vi "OE1311&OE1351_Ethernet_Query Setting.vi"(5 "Connection ID in":refnum<k5>, 7 "Timeout":u32=1000, 11 "Error in (no error)":errorcluster caption="error out（no error）") -> (1 "Input Filter":cluster{"InputCoupling":u8, "InputSource":u8} {"InputSource" items=["A", "B", "Current"]; "InputCoupling" items=["AC", "DC"]}, 2 "Sine Out":T2 {"SineOut Mode" items=["OFF", "Fixed"]}, 3 "System":T1, 6 "Connection ID out":refnum<k5>, 8 "Demodulator":T4 {"Demodulator type_7" items=["Harm", "Arb_Freq"]; "Demodulator type_6" items=["Harm", "Arb_Freq"]; "Demodulator type_5" items=["Harm", "Arb_Freq"]; "Demodulator type_4" items=["Harm", "Arb_Freq"]; "Demodulator type_3" items=["Harm", "Arb_Freq"]; "Demodulator type_2" items=["Harm", "Arb_Freq"]; "Demodulator type_1" items=["Harm", "Arb_Freq"]}, 10 "Output String":string, 12 "Reference Phase":T6 {"External Ref Trigger" items=["TTL Rising Edge", "TTL Fallling Edge", "Sine Zero Crossing"]; "Reference Source" items=["External", "Internal", "Self"]}, 13 "Sensitivity and Filter":T3={"Input Range"=2, "Time Constant(s) "=[], "Low Pass Filter Slope "=1, "Enable Sync Filter "=0} {"Enable Sync Filter" items=["OFF", "ON"]; "Low Pass Filter Slope" items=["6 dB/oct", "12 dB/oct", "18 db/oct", "24 dB/oct", "30 dB/oct", "36 dB/oct", "42 dB/oct", "48 dB/oct"]; "Input Range" items=["5 V/uA", "2 V/uA", "1 V/uA", "500 mV/nA", "200 mV/nA", "100 mV/nA", "50 mV/nA", "20 mV/nA", "10 mV/nA", "5 mV/nA", "2 mV/nA", "1 mV/nA", "500 uV/pA", "200 uV/pA", "100 uV/pA", "50 uV/pA", "20 uV/pA", "10 uV/pA", "5 uV/pA", "2 uV/pA", "1 uV/pA", "500 nV/fA", "200 nV/fA", "100 nV/fA", "50 nV/fA", "20 nV/fA", "10 nV/fA", "5 nV/fA", "2 nV/fA", "1 nV/fA"]}, 14 "Channel Out":T5={"Ch_source_1"=3, "Ch_source_2"=3, "AUX OUT1"=[], "AUX OUT2"=[], "CH1 Offset(%)"=[], "CH2 Offset(%)"=[], "CH1 Expand"=[], "CH2 Expand"=[]} {"Ch_source_2" items=["Fixed", "X", "Y", "R", "Theta", "Xh1", "Yh1", "Rh1", "Theta h1", "Xh2", "Yh2", "Rh2", "Theta h2", "Xh3", "Yh3", "Rh3", "Theta h3", "Rh4", "Xh4", "Yh4", "Theta h4", "Rh5", "Xh5", "Yh5", "Theta h5", "Rh6", "Xh6", "Yh6", "Theta h6", "Rh7", "Xh6", "Yh6", "Theta h7", "X_Noise", "Y_Noise", "Freq", "AuxIn1", "AuxIn2"]; "Ch_source_1" items=["Fixed", "X", "Y", "R", "Theta", "Xh1", "Yh1", "Rh1", "Theta h1", "Xh2", "Yh2", "Rh2", "Theta h2", "Xh3", "Yh3", "Rh3", "Theta h3", "Rh4", "Xh4", "Yh4", "Theta h4", "Rh5", "Xh5", "Yh5", "Theta h5", "Rh6", "Xh6", "Yh6", "Theta h6", "Rh7", "Xh6", "Yh6", "Theta h7", "X_Noise", "Y_Noise", "Freq", "AuxIn1", "AuxIn2"]}, 15 "Error out":errorcluster caption="error out")   [LabVIEW 2011]
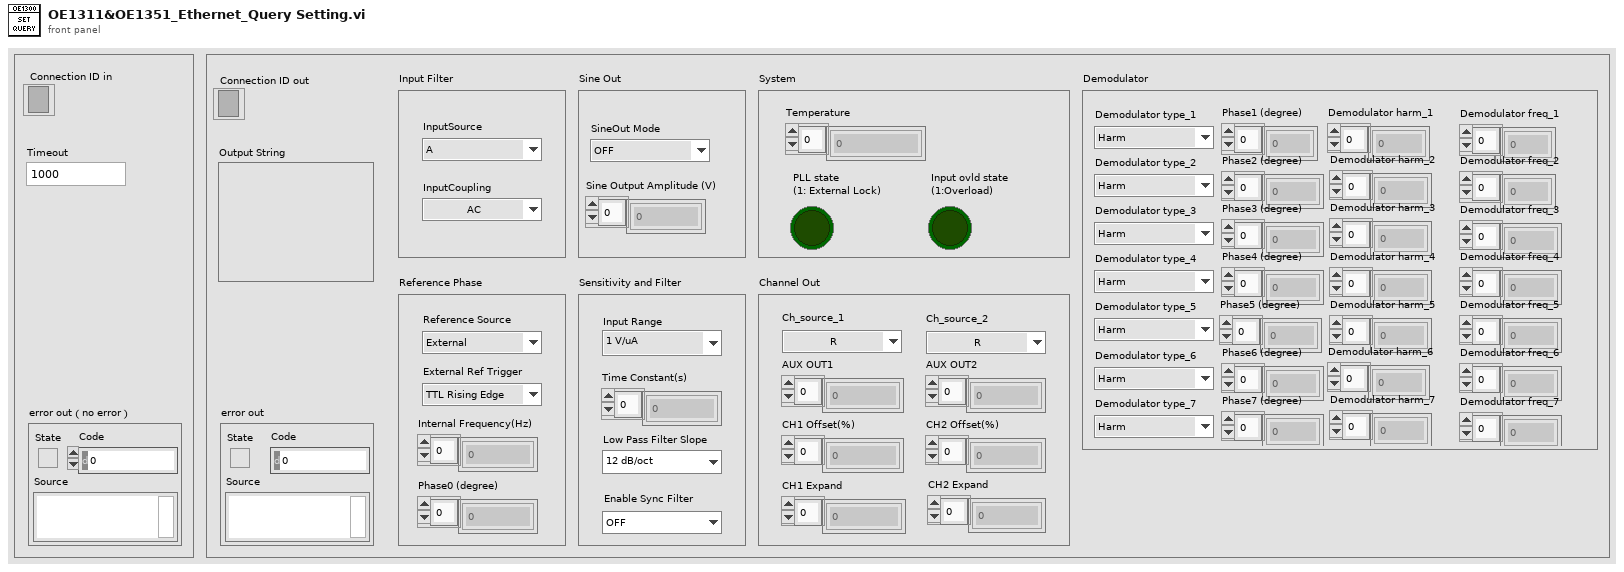
[diagram p1: front panel]
types:
  T1 = cluster{"Temperature":dbl[], "PLL state\n(1: External Lock)":bool, "Input ovld state\n(1:Overload)":bool}
  T2 = cluster{"SineOut Mode":u8, "Sine Output Amplitude (V)":dbl[]}
  T3 = cluster{"Input Range":u8, "Time Constant(s) ":dbl[], "Low Pass Filter Slope ":u8, "Enable Sync Filter ":u8}
  T4 = cluster{"Demodulator type_1":u8, "Demodulator type_2":u8, "Demodulator type_3":u8, "Demodulator type_4":u8, "Demodulator type_5":u8, "Demodulator type_6":u8, "Demodulator type_7":u8, "Phase1 (degree)":dbl[], "Phase2 (degree)":dbl[], "Phase3 (degree)":dbl[], "Phase4 (degree)":sgl[], "Phase5 (degree)":dbl[], "Phase6 (degree)":dbl[], "Phase7 (degree)":dbl[], "Demodulator harm_1":u8[], "Demodulator harm_2":u8[], "Demodulator harm_3":u8[], "Demodulator harm_4":u8[], "Demodulator harm_5":u8[], "Demodulator harm_6":u8[], "Demodulator harm_7":u8[], "Demodulator freq_1":dbl[], "Demodulator freq_2":dbl[], "Demodulator freq_3":dbl[], "Demodulator freq_4":dbl[], "Demodulator freq_5":dbl[], "Demodulator freq_6":dbl[], "Demodulator freq_7":dbl[]}
  T5 = cluster{"Ch_source_1":u8, "Ch_source_2":u8, "AUX OUT1":dbl[], "AUX OUT2":dbl[], "CH1 Offset(%)":dbl[], "CH2 Offset(%)":dbl[], "CH1 Expand":dbl[], "CH2 Expand":dbl[]}
  T6 = cluster{"Phase0 (degree)":dbl[], "Internal Frequency(Hz)":dbl[], "Reference Source":u8, "External Ref Trigger":u8}
  T7 = enum16{"ISRC", "IGND", "ICPL", "ILIN", "PHAS", "FMOD", "RSLP", "FREQ", "SWPT", "SLLM", "SULM", "SSLL", "SSLG", "STLM", "SWRM", "IRNG", "SENS", "RMOD", "OFLT", "OFSL", "SYNC", "DMOD", "HARM", "DARB", "SWVT", "SLVL", "SVLL", "SVUL", "SVSL", "SVSG", "SVTM", "SVRM", "RALL", "SNAP", "OUTP", "OAUX", "COUT", "CAUX", "COFP", "CEXP", "FPOP", "OEXP", "*IDN", "*RST", "OVLD", "INOV", "GNOV", "*PLL", "SSET", "RSET", "AGAN", "APHS", "ARSV", "ASCL", "EQCD", "EQCS", "SPED", "SRAT", "SLEN", "SSLE", "STRG", "SPRM", "STRD", "PAUS", "REST", "SPTS", "TRCA", "TEMP", "RSTU", "IHNZ", "DEQU", "SADD", "ARNG", "CSPE", "ISRCD", "IGNDD", "ICPLD", "ILIND", "PHASD", "FMODD", "RSLPD", "FREQD", "SWPTD", "SLLMD", "SULMD", "SSLLD", "SSLGD", "STLMD", "SWRMD", "SENSD", "RMODD", "OFLTD", "OFSLD", "SYNCD", "HARMD", "EQCDD", "EQCSD", "SNAPD", "OUTPD", "SWVTD", "SLVLD", "SVLLD", "SVULD", "SVSLD", "SVSGD", "SVTMD", "SVRMD", "SVDCD", "ARSVD", "AGAND", "APHSD", "ASCLD", "FPOPD", "CAUXD", "OEXPD", "SPEDD", "SRATD", "SLEND", "SSLED", "STRGD", "SPRMD", "STRDD", "PAUSD", "RESTD", "SPTSD", "TRCAD", "*IDND", "*RSTD", "INOVD", "GNOVD", "*PLLD", "SSETD", "RSETD", "RALLD"}
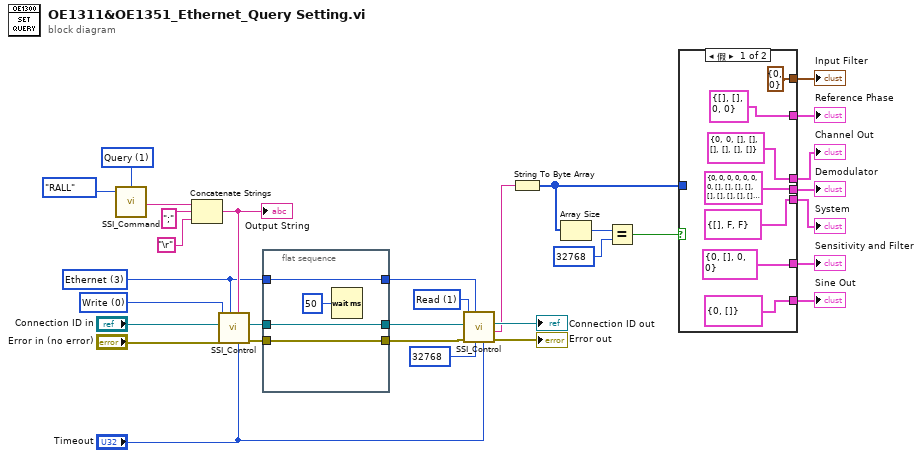
[diagram p0: block diagram]
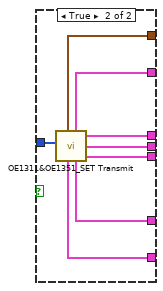
[diagram p2: hidden frame]
diagram:
  w13 = u16 3 items=["USB", "RS232", "GPIB", "Ethernet"] ("Remote Mode")
  w23 = u16 1 items=["Set", "Query"] ("Opera")
  w28 = u16 1 items=["Write", "Read"] ("Control")
  w29 = u16 0 items=["Write", "Read"] ("Control")
  n1 = call "SSI_Command.vi"("Opera"=w23, "Command Type"=T7."RALL") -> ("Output string"=w22:string)  [unwired: 2 in]
  n2 = Concatenate Strings(w22, ";" ("字符串"), "\r") -> (w26:string)
  "Output String" <- w26
  n3 = call "SSI_Control.vi"("Tineout"="Timeout", "Write Buffer"=w26, "Remote Mode"=w13, "Error in (no error)"="Error in (no error)", "Control"=w29, "Connection ID in"="Connection ID in") -> ("Error out"=w16:errorcluster, "Connection ID out"=w15:refnum<k5>)  [unwired: 2 in, 2 out]
  n4 = flat-sequence {
    tunnel: [w36] -> w17
    tunnel: w16 -> [w36]
    tunnel: w15 -> [w35]
    tunnel: [w35] -> w14
    tunnel: [w34] -> w12
    tunnel: w13 -> [w34]
    frame #0 {
      n5 = Wait (ms)(milliseconds to wait=u32 50 ("等待时间（毫秒）")) -> ()  [unwired: 1 out]
    }
  }
  n6 = call "SSI_Control.vi"("Tineout"="Timeout", "Number of bytes"=u32 32768, "Remote Mode"=w12, "Error in (no error)"=w17, "Control"=w28, "Connection ID in"=w14) -> ("Error out"=→"Error out":errorcluster, "Read Buffer"=w19:string, "Connection ID out"=→"Connection ID out":refnum<k5>)  [unwired: 2 in, 1 out]
  n7 = String To Byte Array(string=w19) -> (unsigned byte array=w11:u8[])
  n8 = Array Size(array=w11) -> (size(s)=w10:i32)
  n9 = Equal?(x=w10, y=32768) -> (x = y?=w1:bool)
  n10 = case shown="假" w1 {
    tunnel: w11 -> [_ w51]
    tunnel: [cluster{"InputCoupling":u8, "InputSource":u8} {"InputCoupling"=0, "InputSource"=0} ("Input Filter") w50] -> w8
    tunnel: [T6 {"Phase0 (degree)"=[], "Internal Frequency(Hz)"=[], "Reference Source"=0, "External Ref Trigger"=0} ("Reference Phase") w49] -> w7
    tunnel: [T5 {"Ch_source_1"=0, "Ch_source_2"=0, "AUX OUT1"=[], "AUX OUT2"=[], "CH1 Offset(%)"=[], "CH2 Offset(%)"=[], "CH1 Expand"=[], "CH2 Expand"=[]} ("Channel Out") w48] -> w6
    tunnel: [T4 {"Demodulator type_1"=0, "Demodulator type_2"=0, "Demodulator type_3"=0, "Demodulator type_4"=0, "Demodulator type_5"=0, "Demodulator type_6"=0, "Demodulator type_7"=0, "Phase1 (degree)"=[], "Phase2 (degree)"=[], "Phase3 (degree)"=[], "Phase4 (degree)"=[], "Phase5 (degree)"=[], "Phase6 (degree)"=[], "Phase7 (degree)"=[], "Demodulator harm_1"=[], "Demodulator harm_2"=[], "Demodulator harm_3"=[], "Demodulator harm_4"=[], "Demodulator harm_5"=[], "Demodulator harm_6"=[], "Demodulator harm_7"=[], "Demodulator freq_1"=[], "Demodulator freq_2"=[], "Demodulator freq_3"=[], "Demodulator freq_4"=[], "Demodulator freq_5"=[], "Demodulator freq_6"=[], "Demodulator freq_7"=[]} ("Demodulator") w47] -> w5
    tunnel: [T3 {"Input Range"=0, "Time Constant(s) "=[], "Low Pass Filter Slope "=0, "Enable Sync Filter "=0} ("Sensitivity and Filter") w46] -> w4
    tunnel: [T2 {"SineOut Mode"=0, "Sine Output Amplitude (V)"=[]} ("Sine Out") w45] -> w3
    tunnel: [T1 {"Temperature"=[], "PLL state\n(1: External Lock)"=FALSE, "Input ovld state\n(1:Overload)"=FALSE} ("System") w44] -> w2
    frame False {
    }
    frame True {
      n11 = call "OE1311&OE1351_SET Transmit.vi"("Input Data"=w51) -> ("System"=w44:T1, "Sensitivity and Filter"=w46:T3, "Demodulator"=w47:T4, "Channel Out"=w48:T5, "Reference Phase"=w49:T6, "Sine Out"=w45:T2, "Input Filter"=w50:cluster{"InputCoupling":u8, "InputSource":u8})  [unwired: 3 in]
    }
  }
  "Input Filter" <- w8
  "Reference Phase" <- w7
  "Channel Out" <- w6
  "Demodulator" <- w5
  "Sensitivity and Filter" <- w4
  "Sine Out" <- w3
  "System" <- w2
